vi "http parse function.vi"(9 "handler queue":refnum<queue>, 10 "data in":string, 11 "application request in":T1) -> (2 "abort":bool, 3 "application request out":T1)   [LabVIEW 2016, in "Basic HTTP server.lvclass"]
uses:
  Basic HTTP server.lvclass
  http request.ctl
  http method.ctl
  HTTP headers/http header data.ctl
  HTTP headers/http headers.lvlib
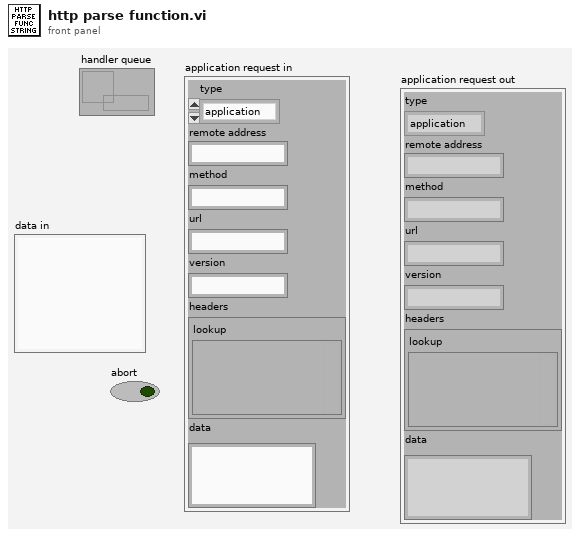
[diagram p1: front panel]
types:
  T1 = typedef "Basic HTTP server.lvclass/http request.ctl" = cluster{"type":T2, "remote address":string, "method":string, "url":string, "version":string, "headers":T3, "data":string}
  T2 = typedef "Basic HTTP server.lvclass/http method.ctl" = enum16{"application", "error", "upgrade", "expect"}
  T3 = typedef "http headers.lvlib/http header data.ctl" = cluster{"lookup":variant}
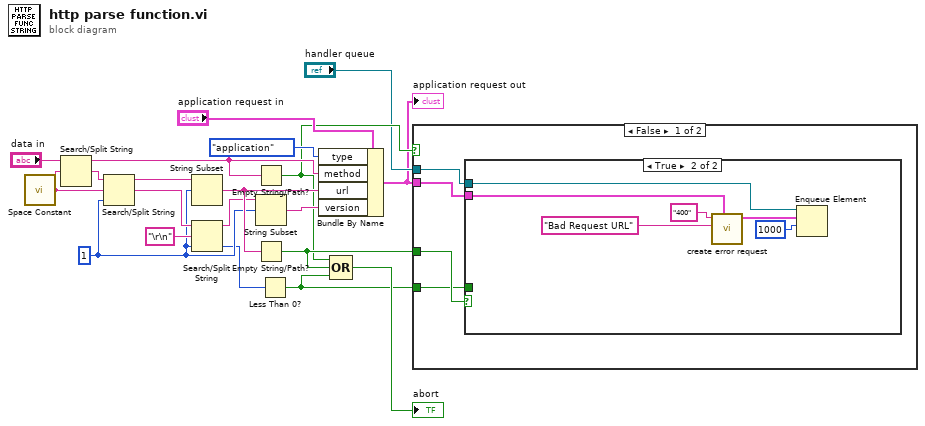
[diagram p0: block diagram]
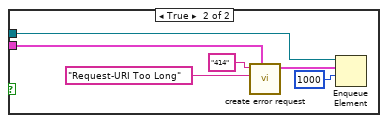
[diagram p3: hidden frame]
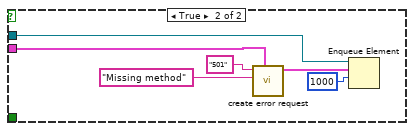
[diagram p4: hidden frame]
diagram:
  w9 = 1 ("offset (0)")
  n1 = call <vilib>:"Space Constant.vi"() -> ("String"=w15:string)
  n2 = Search/Split String(string="data in", search string/char (-)=w15) -> (substring before match=w4:string, match + rest of string=w16:string)  [unwired: 1 in, 1 out]
  n3 = Search/Split String(string=w16, search string/char (-)=w15, offset (0)=w9) -> (substring before match=w14:string, match + rest of string=w12:string)  [unwired: 1 out]
  n4 = String Subset(string=w14, offset (0)=w9) -> (substring=w13:string)  [unwired: 1 in]
  n5 = Search/Split String(string=w12, search string/char (-)="\r\n", offset (0)=w9) -> (substring before match=w10:string, offset of match=w7:i32)  [unwired: 1 out]
  n6 = Empty String/Path?(string/path=w4) -> (empty?=w3:bool)
  n7 = String Subset(string=w10, offset (0)=w9) -> (substring=w8:string)  [unwired: 1 in]
  n8 = Empty String/Path?(string/path=w13) -> (empty?=w18:bool)
  n9 = Less Than 0?(x=w7) -> (x < 0?=w6:bool)
  n10 = Bundle By Name(cluster="application request in", "type"=http_method."application", "method"=w4, "url"=w13, "version"=w8) -> (w1:T1)
  "application request out" <- w1
  n11 = Compound Arithmetic op=OR(w3, w18, w6) -> (→"abort":bool)
  n12 = case shown="False" w3 {
    tunnel: "handler queue" -> [w23 w45]
    tunnel: w18 -> [w24 _]
    tunnel: w6 -> [w22 _]
    tunnel: w1 -> [w21 w40]
    frame False {
      n13 = case shown="True" w24 {
        tunnel: w23 -> [w26 w39]
        tunnel: w22 -> [w27 _]
        tunnel: w21 -> [w25 w34]
        frame False {
          n14 = case shown="False" w27 {
            tunnel: w26 -> [_ w33]
            tunnel: w25 -> [_ w28]
            frame False {
            }
            frame True {
              n15 = call "create error request.vi"("incoming request"=w28, "reason"="Request-URI Too Long" ("status string"), "code"="414") -> ("element"=w32:T1)  [unwired: 8 in]
              n16 = Enqueue Element(queue=w33, element=w32, timeout in ms (-1)=1000) -> ()  [unwired: 1 in, 3 out]
            }
          }
        }
        frame True {
          n17 = call "create error request.vi"("incoming request"=w34, "reason"="Bad Request URL" ("data"), "code"="400" ("method")) -> ("element"=w36:T1)  [unwired: 8 in]
          n18 = Enqueue Element(queue=w39, element=w36, timeout in ms (-1)=1000) -> ()  [unwired: 1 in, 3 out]
        }
      }
    }
    frame True {
      n19 = call "create error request.vi"("incoming request"=w40, "reason"="Missing method" ("data"), "code"="501" ("method")) -> ("element"=w44:T1)  [unwired: 8 in]
      n20 = Enqueue Element(queue=w45, element=w44, timeout in ms (-1)=1000) -> ()  [unwired: 1 in, 3 out]
    }
  }
